vi "Cluster_by_reference.vi"() -> ()   [LabVIEW 2011]
panel:
  in  "Cluster":T1
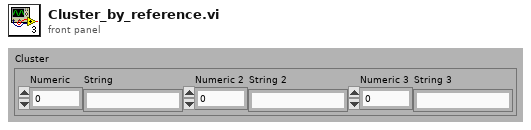
[diagram p1: front panel]
types:
  T1 = cluster{"Numeric":dbl, "String":string, "Numeric 2":dbl, "String 2":string, "Numeric 3":dbl, "String 3":string}
  T2 = enum16{"open", "replace", "create", "open or create", "replace or create", "replace or create with confirmation"}
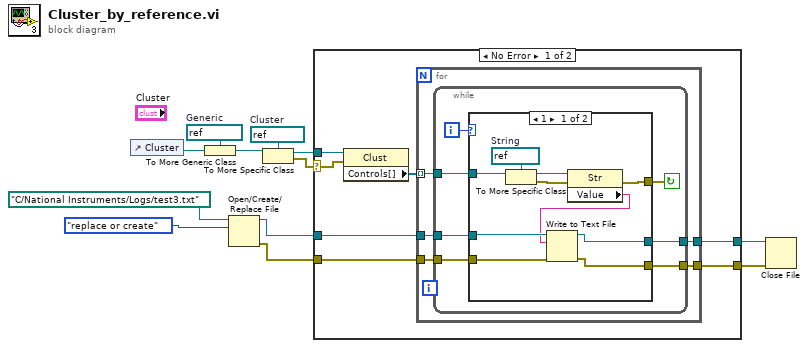
[diagram p0: block diagram]
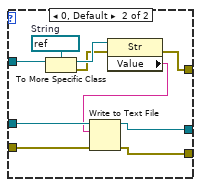
[diagram p2: hidden frame]
diagram:
  w9 = refnum<vi> refnum  # Cluster
  w11 = refnum<vi> refnum  # Generic
  n1 = control-ref of="Cluster"() -> (w12:refnum<vi>)
  n2 = To More Generic Class(target class=w11, reference=w12) -> (generic class reference=w10:refnum<vi>)
  n3 = Open/Create/Replace File(file path (use dialog)=path "C:/National Instruments/Logs/test3.txt" ("base path"), operation (0:open)=T2."replace or create") -> (refnum out=w4:refnum<file>, error out=w3:errorcluster)  [unwired: 4 in, 1 out]
  n4 = To More Specific Class(target class=w9, reference=w10) -> (specific class reference=w8:refnum<vi>, error out=w7:errorcluster)  [unwired: 1 in]
  n5 = case shown="No Error" w7 {
    selector: w7 -> [w18 _]
    tunnel: w8 -> [w19 _]
    tunnel: w4 -> [w16 w53]
    tunnel: w3 -> [w15 w52]
    tunnel: [w14 w53] -> w2
    tunnel: [w13 w52] -> w1
    frame No Error {
      n6 = property class="Clust"(reference=w19, error in=w18) -> ("Controls[]"=w17:refnum<vi>[])  [unwired: 2 out]
      n7 = for {
        tunnel: w17 -> [w24] mode=indexing
        tunnel: w16 -> [w23]
        tunnel: w15 -> [w22]
        tunnel: [w21] -> w14
        tunnel: [w20] -> w13
        n8 = while {
          tunnel: w24 -> [w31]
          tunnel: w23 -> [w28]
          tunnel: w22 -> [w27]
          tunnel: [w26] -> w21
          tunnel: [w25] -> w20
          i -> [w30]
          stop <- w29 continue-if-true
          n9 = case shown="1" w30 {
            tunnel: w31 -> [w41 w51]
            tunnel: [w37 w47] -> w29
            tunnel: w28 -> [w35 w46]
            tunnel: w27 -> [w34 w45]
            tunnel: [w36 w44] -> w26
            tunnel: [w33 w43] -> w25
            frame 1 {
              w40 = refnum<vi> refnum  # String
              n10 = To More Specific Class(target class=w40, reference=w41) -> (specific class reference=w39:refnum<vi>, error out=w38:errorcluster)  [unwired: 1 in]
              n11 = property class="Str"(reference=w39, error in=w38) -> (error out=w37:errorcluster, "Value"=w32:string)  [unwired: 1 out]
              n12 = Write to Text File(file (use dialog)=w35, text=w32, error in=w34) -> (refnum out=w36:refnum<file>, error out=w33:errorcluster)  [unwired: 1 in, 1 out]
            }
            frame 0, Default {
              w50 = refnum<vi> refnum  # String
              n13 = To More Specific Class(target class=w50, reference=w51) -> (specific class reference=w49:refnum<vi>, error out=w48:errorcluster)  [unwired: 1 in]
              n14 = property class="Str"(reference=w49, error in=w48) -> (error out=w47:errorcluster, "Value"=w42:string)  [unwired: 1 out]
              n15 = Write to Text File(file (use dialog)=w46, text=w42, error in=w45) -> (refnum out=w44:refnum<file>, error out=w43:errorcluster)  [unwired: 1 in, 1 out]
            }
          }
        }
      }
    }
    frame Error {
    }
  }
  n16 = Close File(refnum=w2, error in=w1) -> ()  [unwired: 2 out]
